vi "SOLICITAR DATOS DE CONEXION.vi"(5 "MICRO":string, 7 "SE CONECTÓ?":bool, 8 "error in (no error)":errorcluster, 9 "ESTADO ERROR":string, 10 "VISA resource name":refnum<visa-resource-name>) -> (0 "error out":errorcluster)   [LabVIEW 2019, in "MAIN.lvlib"]
doc: "EL MAIN SOLICITA AL MODULO DE CONEXIÓN QUE LE MANDE LAS SIGUIENTES COSAS:\nSESIÓN DE LA CONEXIÓN\nESTADO CONEXIÓN \nESTADO DE ERRORES\nA QUE MICROCONTROLADOR SE CONECTÓ\n_____\nCreated using Delacor QMH Event Scripter 5.0.0.112."
uses:
  MAIN.lvlib
  SOLICITAR DATOS DE CONEXION Argument--cluster.ctl
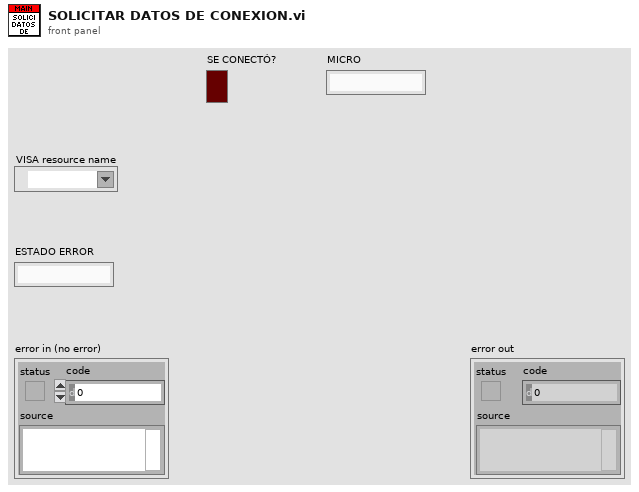
[diagram p1: front panel]
types:
  T1 = typedef "MAIN.lvlib/SOLICITAR DATOS DE CONEXION Argument--cluster.ctl" = cluster{"VISA resource name":refnum<visa-resource-name>, "ESTADO ERROR":string, "SE CONECTÓ?":bool, "MICRO":string}
  T2 = typedef "MAIN.lvlib/Request Events--cluster.ctl" = cluster{"Stop Module":refnum<user-event>, "Show Panel":refnum<user-event>, "Hide Panel":refnum<user-event>, "Get Module Execution Status":refnum<user-event>, "Show Diagram":refnum<user-event>, "START HELPER LOOP":refnum<user-event>, "STOP HELPER LOOP":refnum<user-event>, "SOLICITAR DATOS DE CONEXION":refnum<user-event>}
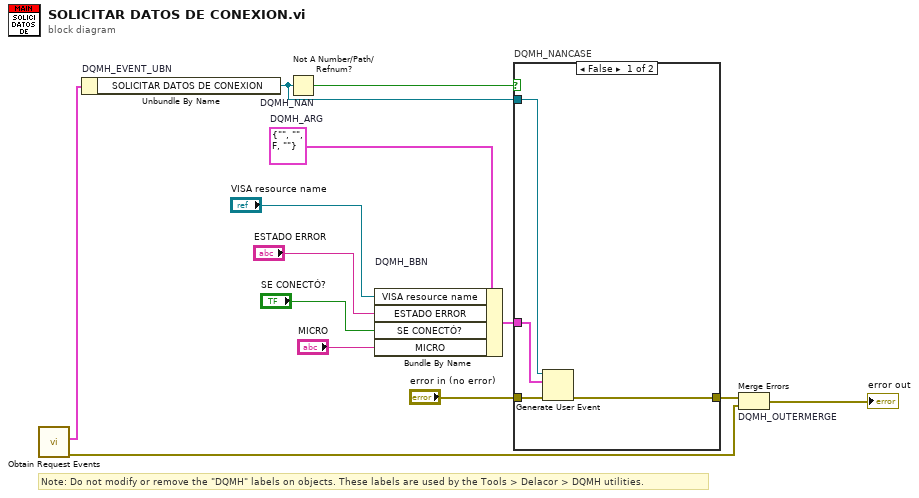
[diagram p0: block diagram]
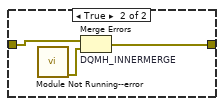
[diagram p2: hidden frame]
diagram:
  w7 = T1 {"VISA resource name"="", "ESTADO ERROR"="", "SE CONECTÓ?"=FALSE, "MICRO"=""}  # DQMH_ARG
  # "Note: Do not modify or remove the \"DQMH\" labels on objects. These labels are used by the Tools > Delacor > DQMH utilities."
  n1 = call "Obtain Request Events.vi"() -> ("error out"=w2:errorcluster, "MAIN Request Events"=w1:T2)  [unwired: 10 in]
  n2 = Unbundle By Name "DQMH_EVENT_UBN"(w1) -> ("SOLICITAR DATOS DE CONEXION"=w9:refnum<user-event>)
  n3 = Not A Number/Path/Refnum? "DQMH_NAN"(number/path/refnum=w9) -> (NaN/Path/Refnum?=w10:bool)
  n4 = Bundle By Name "DQMH_BBN"(cluster=w7, "VISA resource name"="VISA resource name", "ESTADO ERROR"="ESTADO ERROR", "SE CONECTÓ?"="SE CONECTÓ?", "MICRO"="MICRO") -> (w11:T1)
  n5 = case "DQMH_NANCASE" shown="False" w10 {
    tunnel: "error in (no error)" -> [w17 w20]
    tunnel: [w16 w19] -> w8
    tunnel: w9 -> [w15 _]
    tunnel: w11 -> [w14 _]
    frame False {
      n6 = Generate User Event(user event=w15, event data cluster=w14, error in=w17) -> (error out=w16:errorcluster)  [unwired: 1 in, 1 out]
    }
    frame True {
      n7 = call "Module Not Running--error.vi"() -> ("error out"=w18:errorcluster)  [unwired: 11 in]
      n8 = Merge Errors "DQMH_INNERMERGE"(w20, w18) -> (w19:errorcluster)
    }
  }
  n9 = Merge Errors "DQMH_OUTERMERGE"(w8, w2) -> (→"error out":errorcluster)
